vi "Sender vi.vi"() -> ()   [LabVIEW 2014]
panel:
  out "Variable6":T1
  in  "정지":bool
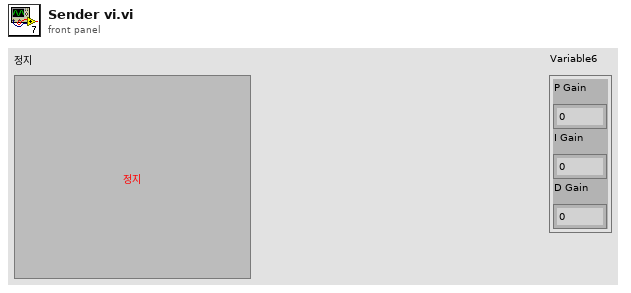
[diagram p1: front panel]
types:
  T1 = cluster{"P Gain":dbl, "I Gain":dbl, "D Gain":dbl}
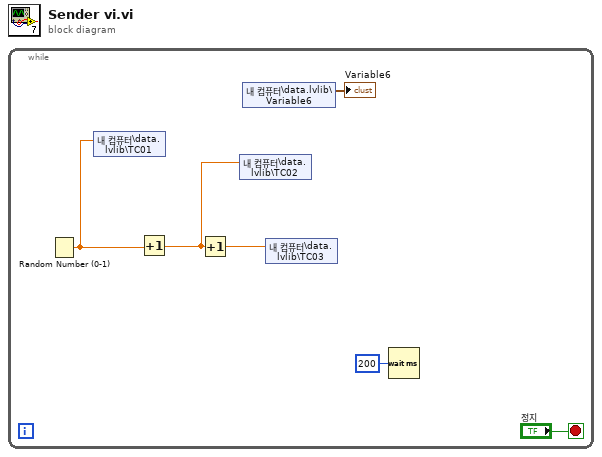
[diagram p0: block diagram]
diagram:
  n1 = while {
    stop <- "정지" stop-if-true
    n2 = Random Number (0-1)() -> (number: 0 to 1=w4:dbl)
    n3 = shared-variable "내 컴퓨터\\data.lvlib\\TC01"(w4) -> ()  [unwired: 1 in, 1 out]
    n4 = Increment(x=w4) -> (x+1=w3:dbl)
    n5 = Increment(x=w3) -> (x+1=w5:dbl)
    n6 = shared-variable "내 컴퓨터\\data.lvlib\\TC02"(w3) -> ()  [unwired: 1 in, 1 out]
    n7 = shared-variable "내 컴퓨터\\data.lvlib\\Variable6"() -> (→"Variable6":T1)  [unwired: 1 in, 1 out]
    n8 = shared-variable "내 컴퓨터\\data.lvlib\\TC03"(w5) -> ()  [unwired: 1 in, 1 out]
    n9 = Wait (ms)(milliseconds to wait=u32 200 ("대기 시간(ms)")) -> ()  [unwired: 1 out]
  }
